vi "comprI+.vi"(2 "I":dbl[][](array[numeric]), 3 "B":dbl[](array[numeric]), 4 "采样点数":i32) -> (0 "I+":dbl[][](array[numeric]), 1 "B+":dbl[](array[numeric]))   [LabVIEW 2018]
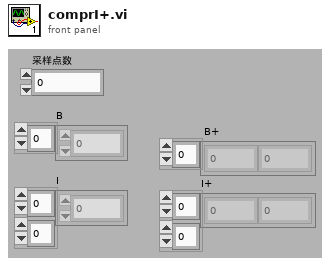
[diagram p1: front panel]
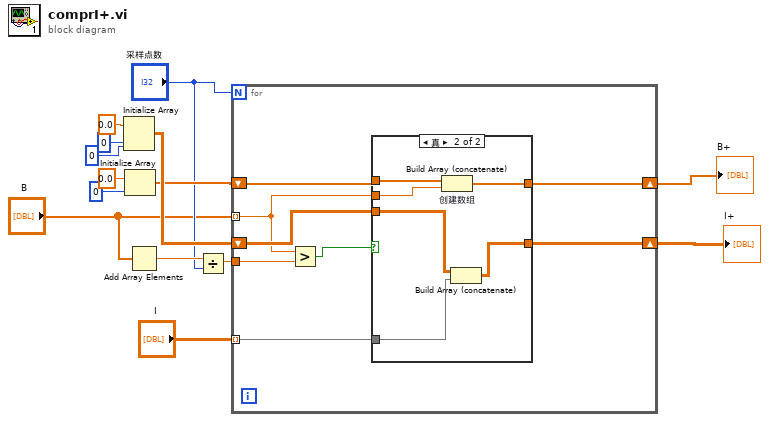
[diagram p0: block diagram]
diagram:
  n1 = Initialize Array(0.0 ("元素"), 0 ("维数大小"), 0 ("维数大小")) -> (w12:dbl[][])
  n2 = Initialize Array(0.0 ("元素"), 0 ("维数大小")) -> (w6:dbl[])
  n3 = Add Array Elements(numeric array="B") -> (sum=w4:dbl)
  n4 = Divide(x=w4, y="采样点数") -> (x/y=w11:dbl)
  n5 = for {
    N: "采样点数" -> [_]
    tunnel: "B" -> [w16] mode=indexing
    shift-right: [w18] -> w9
    shift-left: w12 -> [w22]
    tunnel: w11 -> [w20]
    tunnel: "I" -> [w19] mode=indexing
    shift-right: [w15] -> w5
    shift-left: w6 -> [w17]
    n6 = Greater?(x=w16, y=w20) -> (0:w21:bool)
    n7 = case shown="真" w21 {
      tunnel: w22 -> [w24 w29]
      tunnel: [w24 w30] -> w18
      tunnel: w19 -> [_ w28]
      tunnel: w17 -> [w23 w27]
      tunnel: w16 -> [_ w26]
      tunnel: [w23 w25] -> w15
      frame False {
      }
      frame True {
        n8 = Build Array (concatenate) "创建数组"(w27, w26) -> (w25:dbl[])
        n9 = Build Array (concatenate)(w29, w28) -> (w30:dbl[][])
      }
    }
  }
  "I+" <- w9
  "B+" <- w5
